vi "PixelToUTM.vi"(8 "Resolution of camera in y direction":dbl=1400.0, 9 "Width of camera view in meters":dbl=4.648, 10 "Cluster":cluster{"Y":dbl, "X":dbl}) -> (1 "UTM Location Out":T1)   [LabVIEW 2011]
doc: "Converts the location determined from the camera image to \"UTM Coordinates\", where the reference point is the bottom left of the image. Takes in the pixel coordinates of the boat, returns UTM Coordinates. Can also optionally take in the camera resolution and the width of view."
uses:
  2-RIO/2 Typedefs/UTM Location.ctl
panel:
  out "Meters East":dbl
  out "Meters North":dbl
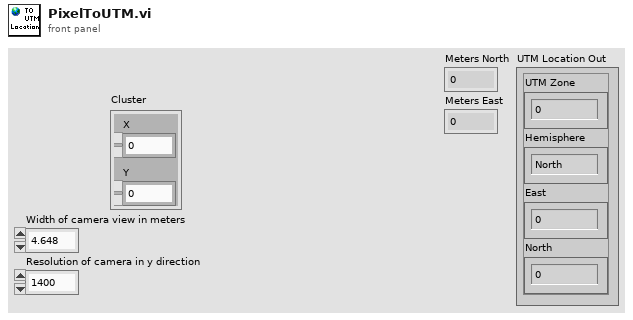
[diagram p1: front panel]
types:
  T1 = typedef "UTM Location.ctl" = cluster{"UTM Zone":dbl, "Hemisphere":enum16{"North", "South"}, "East":dbl, "North":dbl}
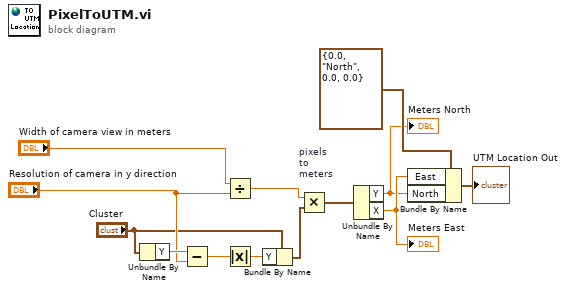
[diagram p0: block diagram]
diagram:
  n1 = Unbundle By Name("Cluster") -> ("Y"=w13:dbl)
  n2 = Subtract(x=w13, y="Resolution of camera in y direction") -> (x-y=w12:dbl)
  n3 = Divide(x="Width of camera view in meters", y="Resolution of camera in y direction") -> (x/y=w1:dbl)
  n4 = Absolute Value(x=w12) -> (abs(x)=w11:dbl)
  n5 = Bundle By Name(cluster="Cluster", "Y"=w11) -> (w3:cluster{"Y":dbl, "X":dbl})
  n6 = Multiply "pixels\nto\nmeters"(x=w1, y=w3) -> (x*y=w10:cluster{"Y":dbl, "X":dbl})
  n7 = Unbundle By Name(w10) -> ("Y"=w7:dbl, "X"=w8:dbl)
  "Meters North" <- w7
  "Meters East" <- w8
  n8 = Bundle By Name(cluster=T1 {"UTM Zone"=0.0, "Hemisphere"=enum."North", "East"=0.0, "North"=0.0} ("UTM Location"), "East"=w8, "North"=w7) -> (→"UTM Location Out":T1)
